vi "Close Report.vi"(0 "reference in":refnum<class "Reporter.lvclass">, 5 "error in (no error)":errorcluster) -> (14 "reference out":refnum<class "Reporter.lvclass">, 19 "error out":errorcluster)   [LabVIEW 2018, in "Reporter.lvclass"]
uses:
  Reporter.lvclass
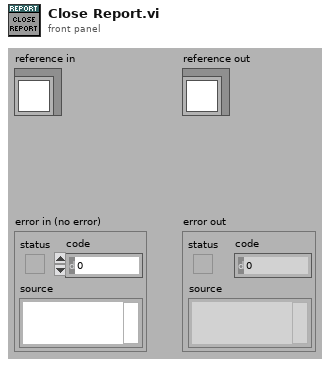
[diagram p1: front panel]
types:
  T1 = typedef "Reporter.lvclass/ObjectAttributes.ctl" = cluster{"LCR":refnum<class "BKP-891 LCR Meter.lvclass">, "PSU":refnum<class "BKP-911x Power Supply.lvclass">, "NI-DAQmx":refnum<class "NI-DAQmx.lvclass">, "Signal List":T2[], "Latest Values":dbl[], "All Latest Values":dbl[], "All Signal List":T2[], "Report Directory":path, "Report File Ref":refnum<file>}
  T2 = typedef "IO Signal List.ctl" = enum16{"Timestamp", "PSU_FB_U_VDC", "PSU_FB_I_AMP", "PSU_FB_W_WATT", "PSU_CMD_U_VDC", "PSU_CMD_I_AMP", "PSU_CMD_OUTPUT", "LCR_PRIMARY", "LCR_SECONDARY", "UV_R_mOhm", "UW_R_mOhm", "VW_R_mOhm", "UV_L_µH", "UW_L_µH", "VW_L_µH", "U_U_VDC", "V_U_VDC", "W_U_VDC", "U_I_AMP", "V_I_AMP", "W_I_AMP", "PWM_CMD_DC_%", "PWM_CMD_VDC", "PWM_CMD_Hz", "PWM_FB_DC_%", "PWM_FB_VDC", "PWM_FB_Hz", "DO_RELAY_U_LCR_A", "DO_RELAY_V_LCR_A", "DO_RELAY_V_LCR_B", "DO_RELAY_W_LCR_B", "DIFF_UV_UW_L_µH", "DIFF_UV_VW_L_µH", "DIFF_UW_VW_L_µH", "DIFF_UV_UW_R_mOhm", "DIFF_UV_VW_R_mOhm", "DIFF_UW_VW_R_mOhm", "DIFF_UV_U_VDC", "DIFF_UW_U_VDC", "DIFF_VW_U_VDC"}
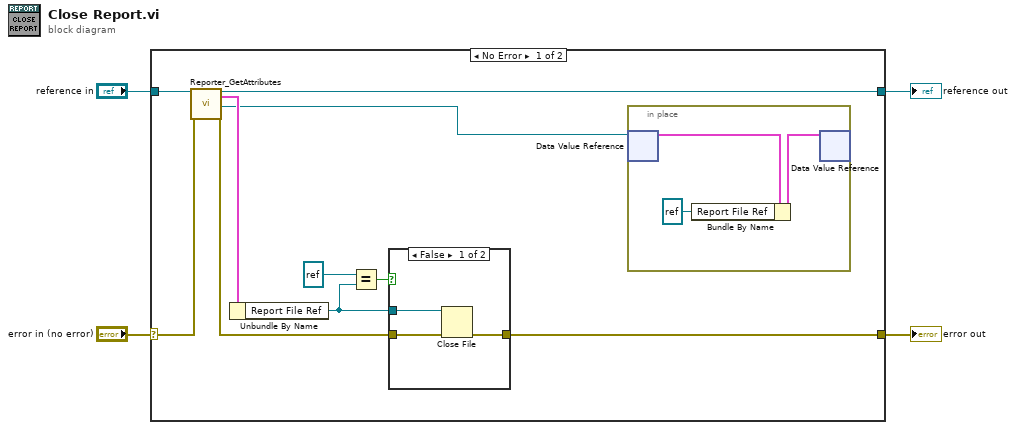
[diagram p0: block diagram]
diagram:
  n1 = case shown="No Error" "error in (no error)" {
    selector: "error in (no error)" -> [w14 w23]
    tunnel: [w9 w23] -> w3
    tunnel: [w11 w22] -> w1
    tunnel: "reference in" -> [w12 w22]
    frame No Error {
      n2 = call "Reporter_GetAttributes.vi"("reference in"=w12, "error in (no error)"=w14) -> ("reference out"=w11:refnum<class "Reporter.lvclass">, "Data"=w13:T1, "DataRef"=w5:refnum<data-value>, "error out"=w10:errorcluster)  [unwired: 14 in]
      n3 = Unbundle By Name(w13) -> ("Report File Ref"=w8:refnum<file>)
      n4 = Equal?(x=refnum<file> refnum, y=w8) -> (x = y?=w6:bool)
      n5 = case shown="False" w6 {
        tunnel: w8 -> [w20 _]
        tunnel: w10 -> [w19 w21]
        tunnel: [w18 w21] -> w9
        frame False {
          n6 = Close File(refnum=w20, error in=w19) -> (error out=w18:errorcluster)  [unwired: 1 out]
        }
        frame True {
        }
      }
      n7 = in-place {
        n8 = in-place-dvr #1(w5) -> (w17:T1)  [unwired: 1 out]
        n9 = Bundle By Name(cluster=w17, "Report File Ref"=refnum<file> refnum) -> (w15:T1)
        n10 = in-place-dvr #1(w15) -> ()  [unwired: 2 out]
      }
    }
    frame Error {
    }
  }
  "error out" <- w3
  "reference out" <- w1
